vi "Simple_Operation.vi"(0 "System no.":i32=1 min=1 step=1, 5 "error in":errorcluster, 12 "Stop refnum":refnum<vi>) -> (19 "error out":errorcluster)   [LabVIEW 2011]
doc: "This VI is runs in a loop until the stop button is pressed, the stop reference is TRUE or an error occures. It lets the operator set the velocity, move the connected axes to relative, absolute or to the home position, and reads the current position continuosly. The diagram shows how to combine the driver and support VIs for these tasks. Use the Help?Show Context Help menu sequence in the LabVIEW environment to display the Context Help window with the VI and control/indicator descriptions.\nRun \" XXXX_Configuration_Setup.vi\" (with XXXX being the PI product number of your system) prior to running this VI. \n\nValid for: C-843, C-843.PM, C-865, C-866, Mercury"
uses:
  Low Level/General command.llb/Global2 (Array).vi
panel:
  in  "Clear":bool
  in  "Define home":bool
  in  "Go home":bool
  in  "Move absolute":bool
  in  "Move relative (+)":bool
  in  "Move relative (-)":bool
  in  "Move":dbl[](array[numeric]) format="%.6f"
  out "Position":dbl[](array[numeric]) format="%.6f"
  in  "Set velocity":bool
  in  "Velocity":dbl[](array[numeric]) format="%.6f"
  in  "stop":bool
  out "Conn. Axes":string[](array[string])
  # "Simple Operation Program"
  # "This VI runs in a loop until the stop button is pressed, the stop reference is TRUE\nor an error occurs. It lets the operator move the connected axes and reads position values. Run \"XXXX_Con-\nfiguration_Setup.vi\" (with XXXX being the PI product number of your system) prior to running this VI."
  # "Command move:"
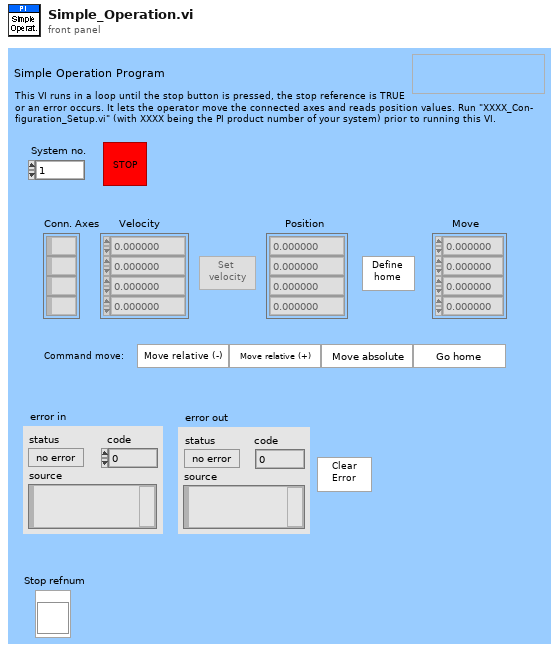
[diagram p1: front panel]
types:
  T1 = typedef "Controller names.ctl" = enum16{"None", "Analog", "C-702", "C-843", "C-843.PM", "C-844", "C-848", "C-865", "C-866", "C-867", "C-880", "E-516", "E-517", "E-710", "E-712", "E-725", "E-753", "E-755", "E-761", "E-816", "E-861", "F-206", "M-840", "M-850", "M-8X0", "Mercury"}
  T2 = cluster{"Conn. axes":string[], "Controller name":T1}[]
  T3 = cluster{"Conn. axes":string[], "Controller name":T1}
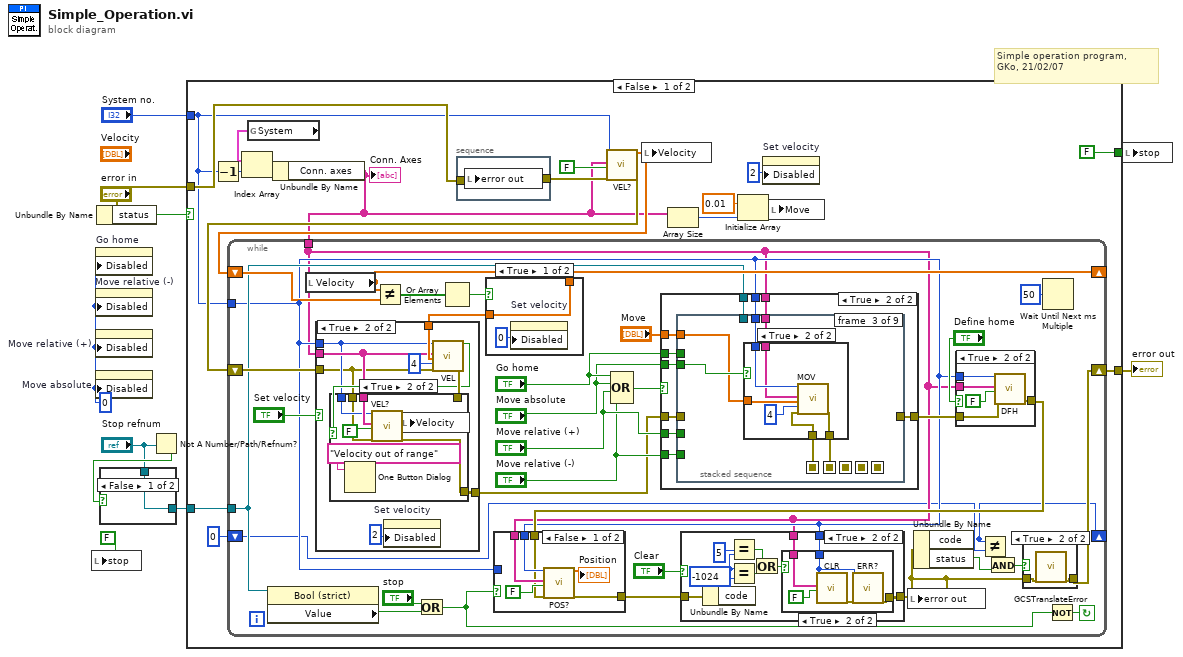
[diagram p0: block diagram]
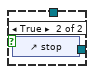
[diagram p2: hidden frame]
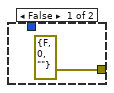
[diagram p5: hidden frame]
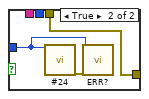
[diagram p6: hidden frame]
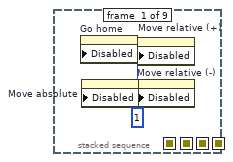
[diagram p8: hidden frame]
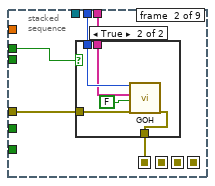
[diagram p9: hidden frame]
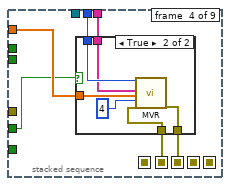
[diagram p12: hidden frame]
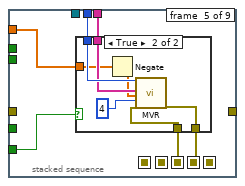
[diagram p14: hidden frame]
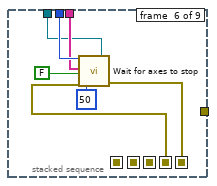
[diagram p16: hidden frame]
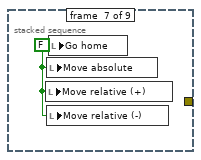
[diagram p17: hidden frame]
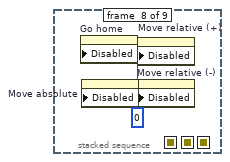
[diagram p18: hidden frame]
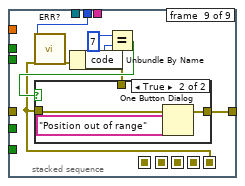
[diagram p19: hidden frame]
diagram:
  w2 = u8 0 ("Disabled")
  # "Simple operation program,\nGKo, 21/02/07"
  n1 = local write "stop"(FALSE ("stop")) -> ()
  n2 = property on="Go home" class="Bool (strict)"("Disabled"=w2) -> ()  [unwired: 2 in, 2 out]
  n3 = property on="Move relative (-)" class="Bool (strict)"("Disabled"=w2) -> ()  [unwired: 2 in, 2 out]
  n4 = property on="Move relative (+)" class="Bool (strict)"("Disabled"=w2) -> ()  [unwired: 2 in, 2 out]
  n5 = property on="Move absolute" class="Bool (strict)"("Disabled"=w2) -> ()  [unwired: 2 in, 2 out]
  n6 = Unbundle By Name("error in") -> ("status"=w9:bool)
  n7 = Not A Number/Path/Refnum?(number/path/refnum="Stop refnum") -> (NaN/Path/Refnum?=w6:bool)
  n8 = case shown="False" w6 {
    tunnel: [w11 w12] -> w5
    tunnel: "Stop refnum" -> [w11 _]
    frame False {
    }
    frame True {
      n9 = control-ref of="stop"() -> (w12:refnum<vi>)
    }
  }
  n10 = case shown="False" w9 {
    tunnel: [w27 w205] -> w8
    tunnel: "error in" -> [w26 w205]
    tunnel: "System no." -> [w17 _]
    tunnel: w5 -> [w24 _]
    tunnel: [FALSE ("stop") FALSE ("stop")] -> w1
    frame False {
      n11 = Decrement(x=w17) -> (x-1=w16:i32)
      n12 = global read "Global2 (Array).vi" "System"() -> (w15:T2)
      n13 = Index Array(array=w15, index=w16) -> (element=w14:T3)
      n14 = Unbundle By Name(w14) -> ("Conn. axes"=w13:string[])
      "Conn. Axes" <- w13
      n15 = stacked-sequence {
        tunnel: w26 -> [w203]
        tunnel: [w203] -> w25
        frame #0 {
          n16 = local write "error out"(w203) -> ()
        }
      }
      n17 = call "VEL?.vi"("System no."=w17, "Axes to query"=w13, "All axes?"=FALSE, "error in"=w25) -> ("Velocity"=w29:dbl[], "error out"=w28:errorcluster)  [unwired: 14 in]
      n18 = while {
        shift-left: 0 ("code") -> [w36]
        shift-right: [w35] -> _
        tunnel: w24 -> [w45]
        tunnel: w13 -> [w37]
        shift-left: w28 -> [w60]
        shift-right: [w39] -> w27
        shift-left: w29 -> [w63]
        shift-right: [w51] -> _
        tunnel: w17 -> [w38]
        stop <- w64 continue-if-true
        n19 = property class="Bool (strict)"(reference=w45) -> ("Value"=w46:bool)  [unwired: 1 in, 2 out]
        n20 = local read "Velocity"() -> (w51:dbl[])
        n21 = Not Equal?(x=w51, y=w63) -> (x != y?=w61:bool[])
        n22 = Or(x="stop", y=w46) -> (x .or. y?=w40:bool)
        n23 = Or Array Elements(Boolean array=w61) -> (logical OR=w62:bool)
        n24 = case shown="True" w62 {
          tunnel: w51 -> [w200 w202]
          tunnel: [w200 w202] -> w50
          frame True {
            n25 = property on="Set velocity" class="Bool"("Disabled"=u8 0 ("Write Attribute")) -> ()  [unwired: 2 in, 2 out]
          }
          frame False {
          }
        }
        n26 = case shown="True" "Set velocity" {
          tunnel: w38 -> [_ w185]
          tunnel: w50 -> [_ w191]
          tunnel: w37 -> [_ w186]
          tunnel: w60 -> [w182 w183]
          tunnel: [w182 w187] -> w48
          frame False {
          }
          frame True {
            n27 = property on="Set velocity" class="Bool"("Disabled"=u8 2 ("Write Attribute")) -> ()  [unwired: 2 in, 2 out]
            n28 = call "VEL.vi"("System no."=w185, "Axes to set"=w186, "Velocity values"=w191, "No.of digits"=i16 4, "error in"=w183) -> ("Controller error"=w188:bool, "error out"=w189:errorcluster)  [unwired: 13 in]
            n29 = case shown="True" w188 {
              tunnel: w189 -> [w192 _]
              tunnel: [w192 w194] -> w187
              tunnel: w186 -> [_ w197]
              tunnel: w185 -> [_ w196]
              tunnel: w183 -> [_ w193]
              frame False {
              }
              frame True {
                n30 = One Button Dialog(message="Velocity out of range") -> ()  [unwired: 1 in, 1 out]
                n31 = call "VEL?.vi"("System no."=w196, "Axes to query"=w197, "All axes?"=FALSE, "error in"=w193) -> ("Velocity"=w195:dbl[], "error out"=w194:errorcluster)  [unwired: 14 in]
                n32 = local write "Velocity"(w195) -> ()
              }
            }
          }
        }
        n33 = Compound Arithmetic op=OR("Go home", "Move absolute", "Move relative (+)", "Move relative (-)") -> (w57:bool)
        n34 = case shown="True" w57 {
          tunnel: "Go home" -> [_ w104]
          tunnel: w38 -> [_ w103]
          tunnel: w37 -> [_ w102]
          tunnel: w48 -> [w94 w101]
          tunnel: "Move absolute" -> [_ w100]
          tunnel: "Move" -> [_ w99]
          tunnel: [w94 w98] -> w44
          tunnel: "Move relative (+)" -> [_ w97]
          tunnel: "Move relative (-)" -> [_ w96]
          tunnel: w45 -> [_ w95]
          frame False {
          }
          frame True {
            n35 = stacked-sequence {
              seq-local: [_ w106 _ _ _ _ _ _ _] -> [_ _ w120 _ _ _ _ _ _]
              seq-local: [_ _ w117 _ _ _ _ _ _] -> [_ _ _ w130 _ _ _ _ _]
              seq-local: [_ _ _ w132 _ _ _ _ _] -> [_ _ _ _ w144 _ _ _ _]
              seq-local: [_ _ _ _ w143 _ _ _ _] -> [_ _ _ _ _ w163 _ _ _]
              seq-local: [_ _ _ _ _ w157 _ _ _] -> [_ _ _ _ _ _ _ _ w166]
              tunnel: w104 -> [_ w110 _ _ _ _ _ _ _]
              tunnel: w103 -> [_ w109 w122 w135 w148 w162 _ _ w172]
              tunnel: w102 -> [_ w108 w121 w134 w147 w161 _ _ _]
              tunnel: w101 -> [_ w107 _ _ _ _ _ _ _]
              tunnel: w100 -> [_ _ w119 _ _ _ _ _ _]
              tunnel: w99 -> [_ _ w118 w133 w146 _ _ _ _]
              tunnel: [_ _ _ _ _ _ _ _ w168] -> w98
              tunnel: w97 -> [_ _ _ w131 _ _ _ _ _]
              tunnel: w96 -> [_ _ _ _ w145 _ _ _ _]
              tunnel: w95 -> [_ _ _ _ _ w158 _ _ _]
              frame #0 {
                w105 = u8 1 ("Disabled")
                n36 = property on="Go home" class="Bool (strict)"("Disabled"=w105) -> ()  [unwired: 2 in, 2 out]
                n37 = property on="Move absolute" class="Bool (strict)"("Disabled"=w105) -> ()  [unwired: 2 in, 2 out]
                n38 = property on="Move relative (+)" class="Bool (strict)"("Disabled"=w105) -> ()  [unwired: 2 in, 2 out]
                n39 = property on="Move relative (-)" class="Bool (strict)"("Disabled"=w105) -> ()  [unwired: 2 in, 2 out]
              }
              frame #1 {
                n40 = case shown="True" w110 {
                  tunnel: w109 -> [_ w116]
                  tunnel: w108 -> [_ w115]
                  tunnel: w107 -> [w111 w113]
                  tunnel: [w111 w112] -> w106
                  frame False {
                  }
                  frame True {
                    n41 = call "GOH.vi"("System no."=w116, "GOH axes"=w115, "All axes?"=FALSE, "error in"=w113) -> ("error out"=w112:errorcluster)  [unwired: 15 in]
                  }
                }
              }
              frame #2 {
                n42 = case shown="True" w119 {
                  tunnel: w122 -> [_ w129]
                  tunnel: w121 -> [_ w128]
                  tunnel: w120 -> [w123 w126]
                  tunnel: w118 -> [_ w125]
                  tunnel: [w123 w124] -> w117
                  frame False {
                  }
                  frame True {
                    n43 = call "MOV.vi"("System no."=w129, "Axes to move"=w128, "Position values"=w125, "No.of digits"=i16 4, "error in"=w126) -> ("error out"=w124:errorcluster)  [unwired: 14 in]
                  }
                }
              }
              frame #3 {
                n44 = case shown="True" w131 {
                  tunnel: w135 -> [_ w142]
                  tunnel: w134 -> [_ w141]
                  tunnel: w133 -> [_ w140]
                  tunnel: [w136 w138] -> w132
                  tunnel: w130 -> [w136 w137]
                  frame False {
                  }
                  frame True {
                    n45 = call "MVR.vi"("System no."=w142, "Axes to move"=w141, "Position values"=w140, "No.of digits"=i16 4, "error in"=w137) -> ("error out"=w138:errorcluster)  [unwired: 14 in]
                  }
                }
              }
              frame #4 {
                n46 = case shown="True" w145 {
                  tunnel: w148 -> [_ w156]
                  tunnel: w147 -> [_ w155]
                  tunnel: w146 -> [_ w153]
                  tunnel: w144 -> [w149 w151]
                  tunnel: [w149 w150] -> w143
                  frame False {
                  }
                  frame True {
                    n47 = Negate(x=w153) -> (-x=w152:dbl[])
                    n48 = call "MVR.vi"("System no."=w156, "Axes to move"=w155, "Position values"=w152, "No.of digits"=i16 4, "error in"=w151) -> ("error out"=w150:errorcluster)  [unwired: 14 in]
                  }
                }
              }
              frame #5 {
                n49 = call "Wait for axes to stop.vi"("System no."=w162, "Axes to wait for"=w161, "With status bit polling?"=FALSE, "error in"=w163, "Polling cycle time, ms"=u32 50, "Stop refnum"=w158) -> ("error out"=w157:errorcluster)  [unwired: 12 in, 1 out]
              }
              frame #6 {
                w164 = FALSE ("Go home")
                n50 = local write "Move relative (+)"(w164) -> ()
                n51 = local write "Move absolute"(w164) -> ()
                n52 = local write "Move relative (-)"(w164) -> ()
                n53 = local write "Go home"(w164) -> ()
              }
              frame #7 {
                w165 = u8 0 ("Disabled")
                n54 = property on="Go home" class="Bool (strict)"("Disabled"=w165) -> ()  [unwired: 2 in, 2 out]
                n55 = property on="Move absolute" class="Bool (strict)"("Disabled"=w165) -> ()  [unwired: 2 in, 2 out]
                n56 = property on="Move relative (+)" class="Bool (strict)"("Disabled"=w165) -> ()  [unwired: 2 in, 2 out]
                n57 = property on="Move relative (-)" class="Bool (strict)"("Disabled"=w165) -> ()  [unwired: 2 in, 2 out]
              }
              frame #8 {
                n58 = call "ERR?.vi"("System no."=w172, "error in"=w166) -> ("error out"=w167:errorcluster)  [unwired: 16 in, 1 out]
                n59 = Unbundle By Name(w167) -> ("code"=w170:i32)
                n60 = Equal?(x=7 ("y"), y=w170) -> (x = y?=w169:bool)
                n61 = case shown="True" w169 {
                  tunnel: [w173 w174] -> w168
                  tunnel: w167 -> [w173 _]
                  tunnel: w166 -> [_ w174]
                  frame False {
                  }
                  frame True {
                    n62 = One Button Dialog(message="Position out of range") -> ()  [unwired: 1 in, 1 out]
                  }
                }
              }
            }
          }
        }
        n63 = case shown="True" "Define home" {
          tunnel: w38 -> [_ w181]
          tunnel: w37 -> [_ w180]
          tunnel: w44 -> [w176 w178]
          tunnel: [w176 w177] -> w43
          frame False {
          }
          frame True {
            n64 = call "DFH.vi"("System no."=w181, "DFH axes"=w180, "All axes?"=FALSE, "error in"=w178) -> ("error out"=w177:errorcluster)  [unwired: 15 in]
          }
        }
        n65 = case shown="False" w40 {
          tunnel: w38 -> [_ w92]
          tunnel: w37 -> [w88 _]
          tunnel: w38 -> [w87 _]
          tunnel: w43 -> [w86 w91]
          tunnel: [w85 w91] -> w41
          frame False {
            n66 = call "POS?.vi"("System no."=w87, "Axes to query"=w88, "All axes?"=FALSE, "error in"=w86) -> ("Position"=→"Position":dbl[], "error out"=w85:errorcluster)  [unwired: 14 in]
          }
          frame True {
            n67 = call "#24.vi"("System no."=w92) -> ("error out"=w93:errorcluster)  [unwired: 18 in]
            n68 = call "ERR?.vi"("System no."=w92, "error in"=w93) -> ()  [unwired: 16 in, 2 out]
          }
        }
        n69 = case shown="True" "Clear" {
          tunnel: [w68 w71] -> w32
          tunnel: w41 -> [w68 w75]
          tunnel: w38 -> [_ w70]
          tunnel: w37 -> [_ w69]
          frame False {
          }
          frame True {
            n70 = Unbundle By Name(w75) -> ("code"=w76:i32)
            n71 = Equal?(x=5 ("y"), y=w76) -> (x = y?=w74:bool)
            n72 = Equal?(x=w76, y=-1024) -> (x = y?=w72:bool)
            n73 = Or(x=w74, y=w72) -> (x .or. y?=w73:bool)
            n74 = case shown="True" w73 {
              tunnel: [errorcluster {"status"=FALSE, "code"=0, "source"=""} ("error out") w83] -> w71
              tunnel: w70 -> [_ w82]
              tunnel: w69 -> [_ w81]
              frame False {
              }
              frame True {
                n75 = call "CLR.vi"("System no."=w82, "CLR axes"=w81, "All axes?"=FALSE) -> ("error out"=w84:errorcluster)  [unwired: 16 in]
                n76 = call "ERR?.vi"("System no."=w82, "error in"=w84) -> ("error out"=w83:errorcluster)  [unwired: 16 in, 1 out]
              }
            }
          }
        }
        n77 = local write "error out"(w32) -> ()
        n78 = Unbundle By Name(w32) -> ("code"=w35:i32, "status"=w31:bool)
        n79 = Not Equal?(x=w35, y=w36) -> (x != y?=w34:bool)
        n80 = And(x=w34, y=w31) -> (x .and. y?=w33:bool)
        n81 = case shown="True" w33 {
          tunnel: w32 -> [w65 w67]
          tunnel: [w65 w66] -> w39
          frame False {
          }
          frame True {
            n82 = call "GCSTranslateError.vi"("error in"=w67) -> ("error out"=w66:errorcluster)  [unwired: 16 in, 2 out]
          }
        }
        n83 = Wait Until Next ms Multiple(millisecond multiple=u32 50) -> ()  [unwired: 1 out]
        n84 = Not(x=w40) -> (.not. x?=w64:bool)
      }
      n85 = local write "Velocity"(w29) -> ()
      n86 = Array Size(array=w13) -> (size(s)=w21:i32)
      n87 = Initialize Array(0.01 ("Move"), w21) -> (w20:dbl[])
      n88 = property on="Set velocity" class="Bool"("Disabled"=u8 2 ("Write Attribute")) -> ()  [unwired: 2 in, 2 out]
      n89 = local write "Move"(w20) -> ()
    }
    frame True {
    }
  }
  "error out" <- w8
  n90 = local write "stop"(w1) -> ()
